vi "Konfig Recipes.vi"() -> ()   [LabVIEW 2020, in "FT-IR.lvlib"]
uses:
  FT-IR.lvlib
  Visualisierungs Elemente/Checkbox(boolsch).ctl
  System Einstellungen V2/Aktioen FGV System.ctl
  Aktion FGV Rezepte wechseln.ctl
  AK-manuell.ctl
  Allgemein/allgemeine Sub-VIs.lvlib
  TOOLweb Interface Library/TOOLweb Interface.lvlib
  System Einstellungen V2/System Einstellungen V2.lvlib
panel:
  in  "AK Konfig aktive":T1 caption="AK Konfiguration für Rezeptwechsel deaktiviert"
  in  "laden":bool caption="Stopp"
  in  "Natural Gas":u16(ring) caption="Natural Gas:"
  in  "Gasoline":u16(ring) caption="Gasoline:"
  in  "Diesel":u16(ring) caption="Diesel:"
  in  "Rezepte:":u16(ring)
  in  "Stopp":bool
  # "FT-IR Rezept wechsel"
  # "AK Konfiguration"
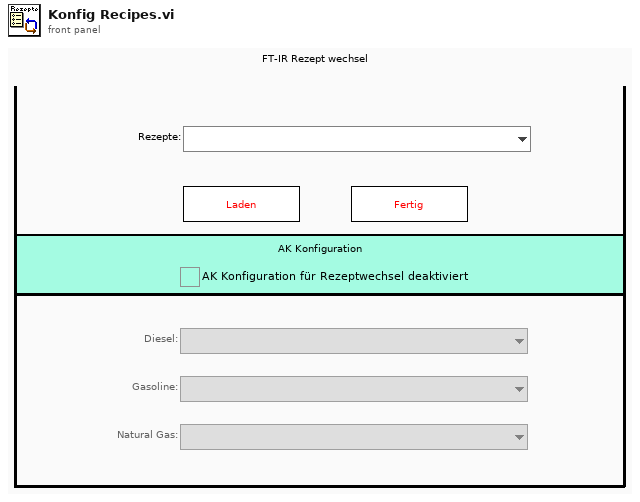
[diagram p1: front panel]
types:
  T1 = typedef "Checkbox(boolsch).ctl" = bool
  T2 = enum8{"Enabled", "Disabled", "Disabled and Grayed Out"}
  T3 = typedef "System Einstellungen V2.lvlib/Aktioen FGV System.ctl" = enum16{"lesen", "laden", "speichern", "Optionen schreiben", "Zeitstempel", "Reset BMP", "Reset SQP", "Wartung", "Werkseinstellung"}
  T4 = typedef "FT-IR.lvlib/AK-manuell.ctl" = enum16{"manuell", "Diesel", "CNG", "Gasoline"}
  T5 = typedef "FT-IR.lvlib/Aktion FGV Rezepte wechseln.ctl" = enum16{"lesen", "Rezepte", "Rezeptindex", "Diesel", "Gasoline", "NCG", "laden", "speichern", "AK/Man"}
  T6 = typedef "System Einstellungen V2.lvlib/Optionen.ctl" = cluster{"Störmeldep.":bool, "Betriebszustände":bool, "AK in ppm":bool, "log Cal-Gas":bool, "log 0-Gas":bool, "Durchflusssensor 0-5V":bool, "PNS?":bool, "Mit N2 spülen":bool, "TRE08":bool, "Amium 10-Fach":bool, "Verticale Scrollbar aktiv":bool, "Loggingtakt":bool, "AK Rezeptwechsel gleich wie MKS":bool, "NG ECO":bool}
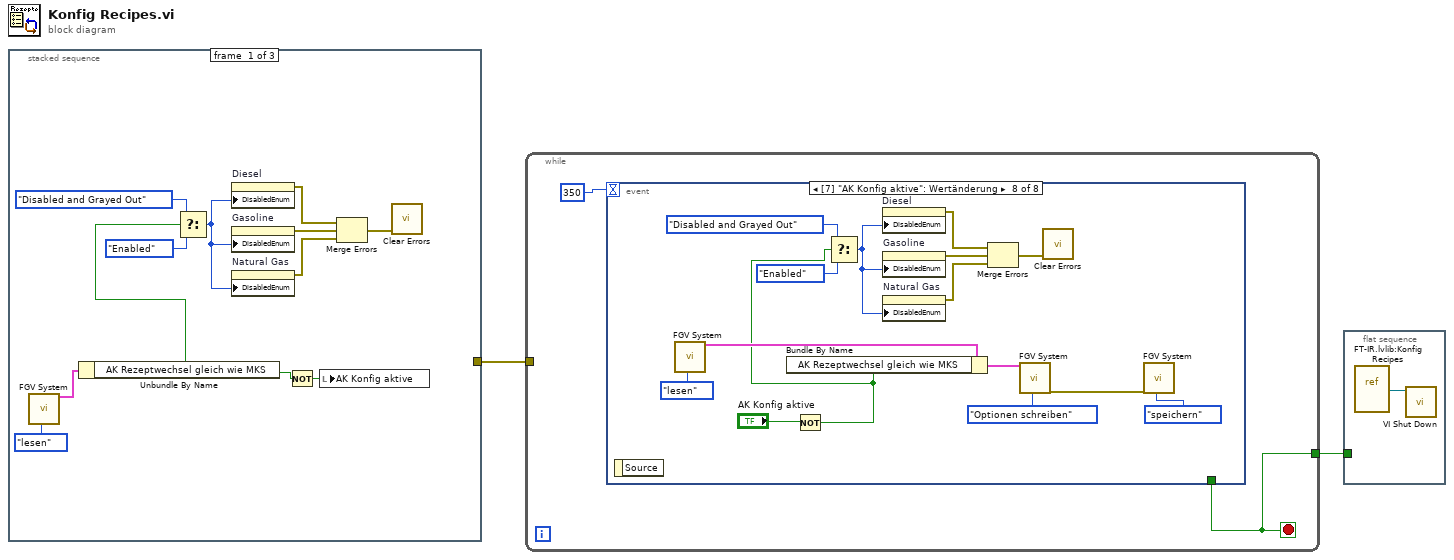
[diagram p0: block diagram]
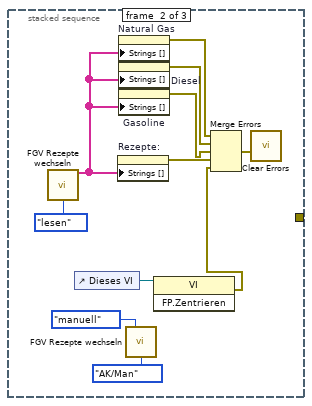
[diagram p2: hidden frame]
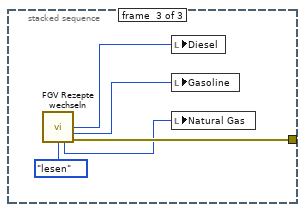
[diagram p3: hidden frame]
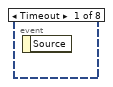
[diagram p4: hidden frame]
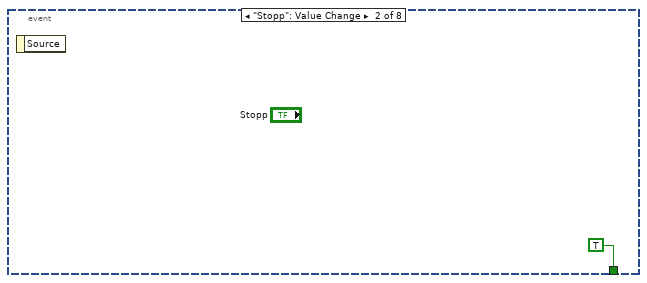
[diagram p5: hidden frame]
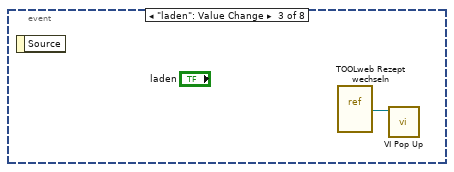
[diagram p6: hidden frame]
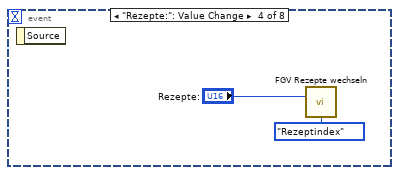
[diagram p7: hidden frame]
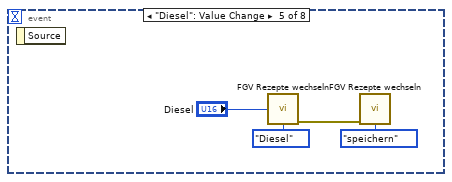
[diagram p8: hidden frame]
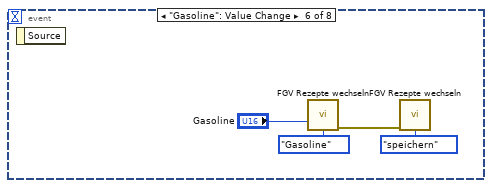
[diagram p9: hidden frame]
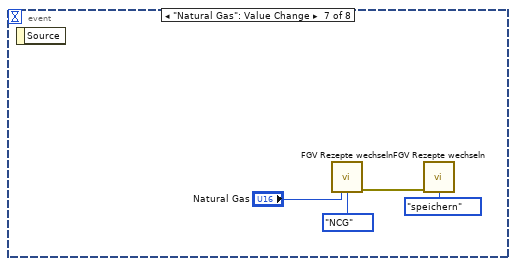
[diagram p10: hidden frame]
diagram:
  n1 = stacked-sequence {
    tunnel: [_ _ w28] -> w1
    frame #0 {
      n2 = call "FGV System.vi"("Aktionen"=Aktioen_FGV_System."lesen") -> ("Optionen"=w13:T6)  [unwired: 12 in, 6 out]
      n3 = Unbundle By Name(w13) -> ("AK Rezeptwechsel gleich wie MKS"=w4:bool)
      n4 = Select(t=T2."Disabled and Grayed Out" ("Deaktiviert"), s=w4, f=T2."Enabled" ("Deaktiviert")) -> (s? t:f=w5:T2)
      n5 = property on="Diesel" class="Ring (strikt)"("DisabledEnum"=w5) -> (error out=w9:errorcluster)  [unwired: 2 in, 1 out]
      n6 = property on="Gasoline" class="Ring (strikt)"("DisabledEnum"=w5) -> (error out=w10:errorcluster)  [unwired: 2 in, 1 out]
      n7 = property on="Natural Gas" class="Ring (strikt)"("DisabledEnum"=w5) -> (error out=w11:errorcluster)  [unwired: 2 in, 1 out]
      n8 = Not(x=w4) -> (.not. x?=w3:bool)
      n9 = local write "AK Konfig aktive"(w3) -> ()
      n10 = Merge Errors(w9, w10, w11) -> (w8:errorcluster)
      n11 = call <vilib>:"Clear Errors.vi"("error in (no error)"=w8) -> ()  [unwired: 5 in, 2 out]
    }
    frame #1 {
      n12 = call "FGV Rezepte wechseln.vi"("Aktion"=Aktion_FGV_Rezepte_wechseln."lesen") -> ("Rezepte"=w16:string[])  [unwired: 8 in, 6 out]
      n13 = control-ref of="Dieses VI"() -> (w22:refnum<vi>)
      n14 = property on="Rezepte:" class="Ring (strikt)"("Strings []"=w16) -> (error out=w23:errorcluster)  [unwired: 2 in, 1 out]
      n15 = property on="Natural Gas" class="Ring (strikt)"("Strings []"=w16) -> (error out=w19:errorcluster)  [unwired: 2 in, 1 out]
      n16 = property on="Diesel" class="Ring (strikt)"("Strings []"=w16) -> (error out=w18:errorcluster)  [unwired: 2 in, 1 out]
      n17 = property on="Gasoline" class="Ring (strikt)"("Strings []"=w16) -> (error out=w17:errorcluster)  [unwired: 2 in, 1 out]
      n18 = call "FGV Rezepte wechseln.vi"("AK/man"=AK-manuell."manuell", "Aktion"=Aktion_FGV_Rezepte_wechseln."AK/Man") -> ()  [unwired: 7 in, 7 out]
      n19 = invoke class="VI" method="FP.Zentrieren"(reference=w22) -> (error out=w20:errorcluster)  [unwired: 2 in, 2 out]
      n20 = Merge Errors(w19, w18, w17, w23, w20) -> (w21:errorcluster)
      n21 = call <vilib>:"Clear Errors.vi"("error in (no error)"=w21) -> ()  [unwired: 5 in, 2 out]
    }
    frame #2 {
      n22 = call "FGV Rezepte wechseln.vi"("Aktion"=Aktion_FGV_Rezepte_wechseln."lesen") -> ("Diesel"=w27:u16, "Gasoline"=w26:u16, "Natural Gas"=w25:u16, "error out"=w28:errorcluster)  [unwired: 8 in, 3 out]
      n23 = local write "Diesel"(w27) -> ()
      n24 = local write "Gasoline"(w26) -> ()
      n25 = local write "Natural Gas"(w25) -> ()
    }
  }
  n26 = while {
    tunnel: [w30] -> w2
    tunnel: w1 -> [_]
    stop <- w30 stop-if-true
    n27 = event shown="[7] \"AK Konfig aktive\": Wertänderung" {
      selector: _ -> [_ _ _ _ _ _ _ _]
      dyn-events: _ -> [_ _ _ _ _ _ _ _]
      timeout: 350 -> [_ _ _ _ _ _ _ _]
      tunnel: [_ TRUE _ _ _ _ _ _] -> w30
      event Timeout {
        n28 = event-data() -> ()  [unwired: 1 in, 1 out]
      }
      event "Stopp": Value Change {
        n29 = event-data() -> ()  [unwired: 1 in, 1 out]
      }
      event "laden": Value Change {
        n30 = event-data() -> ()  [unwired: 1 in, 1 out]
        n31 = vi-ref "TOOLweb Rezept wechseln.vi"() -> (w33:refnum<vi>)
        n32 = call "VI Pop Up.vi"("VI Referenz"=w33) -> ()  [unwired: 10 in, 1 out]
      }
      event "Rezepte:": Value Change {
        n33 = event-data() -> ()  [unwired: 1 in, 1 out]
        n34 = call "FGV Rezepte wechseln.vi"("Rezeptindex"="Rezepte:", "Aktion"=Aktion_FGV_Rezepte_wechseln."Rezeptindex") -> ()  [unwired: 7 in, 7 out]
      }
      event "Diesel": Value Change {
        n35 = event-data() -> ()  [unwired: 1 in, 1 out]
        n36 = call "FGV Rezepte wechseln.vi"("Diesel"="Diesel", "Aktion"=Aktion_FGV_Rezepte_wechseln."Diesel") -> ("error out"=w36:errorcluster)  [unwired: 7 in, 6 out]
        n37 = call "FGV Rezepte wechseln.vi"("error in (no error)"=w36, "Aktion"=Aktion_FGV_Rezepte_wechseln."speichern") -> ()  [unwired: 7 in, 7 out]
      }
      event "Gasoline": Value Change {
        n38 = event-data() -> ()  [unwired: 1 in, 1 out]
        n39 = call "FGV Rezepte wechseln.vi"("Gasoline"="Gasoline", "Aktion"=Aktion_FGV_Rezepte_wechseln."Gasoline") -> ("error out"=w41:errorcluster)  [unwired: 7 in, 6 out]
        n40 = call "FGV Rezepte wechseln.vi"("error in (no error)"=w41, "Aktion"=Aktion_FGV_Rezepte_wechseln."speichern") -> ()  [unwired: 7 in, 7 out]
      }
      event "Natural Gas": Value Change {
        n41 = event-data() -> ()  [unwired: 1 in, 1 out]
        n42 = call "FGV Rezepte wechseln.vi"("Natural Gas"="Natural Gas", "Aktion"=Aktion_FGV_Rezepte_wechseln."NCG") -> ("error out"=w45:errorcluster)  [unwired: 7 in, 6 out]
        n43 = call "FGV Rezepte wechseln.vi"("error in (no error)"=w45, "Aktion"=Aktion_FGV_Rezepte_wechseln."speichern") -> ()  [unwired: 7 in, 7 out]
      }
      event Value Change {
        n44 = event-data() -> ()  [unwired: 1 in, 1 out]
        n45 = call "FGV System.vi"("Aktionen"=Aktioen_FGV_System."lesen") -> ("Optionen"=w52:T6)  [unwired: 12 in, 6 out]
        n46 = Not(x="AK Konfig aktive") -> (.not. x?=w48:T1)
        n47 = Bundle By Name(cluster=w52, "AK Rezeptwechsel gleich wie MKS"=w48) -> (w51:T6)
        n48 = Select(t=T2."Disabled and Grayed Out" ("Deaktiviert"), s=w48, f=T2."Enabled" ("Deaktiviert")) -> (s? t:f=w62:T2)
        n49 = property on="Diesel" class="Ring (strikt)"("DisabledEnum"=w62) -> (error out=w58:errorcluster)  [unwired: 2 in, 1 out]
        n50 = property on="Gasoline" class="Ring (strikt)"("DisabledEnum"=w62) -> (error out=w57:errorcluster)  [unwired: 2 in, 1 out]
        n51 = property on="Natural Gas" class="Ring (strikt)"("DisabledEnum"=w62) -> (error out=w56:errorcluster)  [unwired: 2 in, 1 out]
        n52 = Merge Errors(w58, w57, w56) -> (w59:errorcluster)
        n53 = call "FGV System.vi"("Optionen"=w51, "Aktionen"=Aktioen_FGV_System."Optionen schreiben") -> ("error out"=w49:errorcluster)  [unwired: 11 in, 6 out]
        n54 = call <vilib>:"Clear Errors.vi"("error in (no error)"=w59) -> ()  [unwired: 5 in, 2 out]
        n55 = call "FGV System.vi"("error in (no error)"=w49, "Aktionen"=Aktioen_FGV_System."speichern") -> ()  [unwired: 11 in, 7 out]
      }
    }
  }
  n56 = flat-sequence {
    tunnel: w2 -> [_]
    frame #0 {
      n57 = vi-ref "FT-IR.lvlib:Konfig Recipes.vi"() -> (w63:refnum<vi>)
      n58 = call "VI Shut Down.vi"("VI Referenz"=w63) -> ()  [unwired: 11 in]
    }
  }
